vi "Invalid DLS Profile.vi"(0 "GEA2 Reference In":refnum<k24>, 1 "Shift To":enum16{"Spin", "Agitate"}(ring), 2 "Input Bit":T2, 5 "GEA Inputs":T4={"Source"=228, "Destination"=35} {"Destination" format="%.0x"; "Source" format="%.0x"}, 7 "Standalone?":bool, 11 "Error In":errorcluster, 12 "Action":enum16{"Lock", "Unlock"}(ring), 13 "Co-efficient Data":T1) -> (4 "GEA2 Reference Out":refnum<k24>, 10 "Report Text":string, 14 "Pass/Fail":bool, 15 "Error Out":errorcluster)   [LabVIEW 2016, in "TL27.lvlib"]
uses:
  Projects/TL27.lvlib
  C:/Automation/DLLs/PC Dot Net/GeaCommunication.dll
  Common/LabVIEW GEA2 Toolkit/LabVIEW_GEA2_Toolkit.lvlibp/type defs/Source_Destination.ctl
  Control/DLS ERD Data.ctl
  Valew Common/type defs/Drive Cycle Engine Request State.ctl
  Common/LabVIEW GEA2 Toolkit/LabVIEW_GEA2_Toolkit.lvlibp/type defs/ERD Read Data In.ctl
  Common/LabVIEW GEA2 Toolkit/LabVIEW_GEA2_Toolkit.lvlibp/type defs/Data Type.ctl
  Common/LabVIEW GEA2 Toolkit/LabVIEW_GEA2_Toolkit.lvlibp
panel:
  out "R1_DLS ERD Data":T3
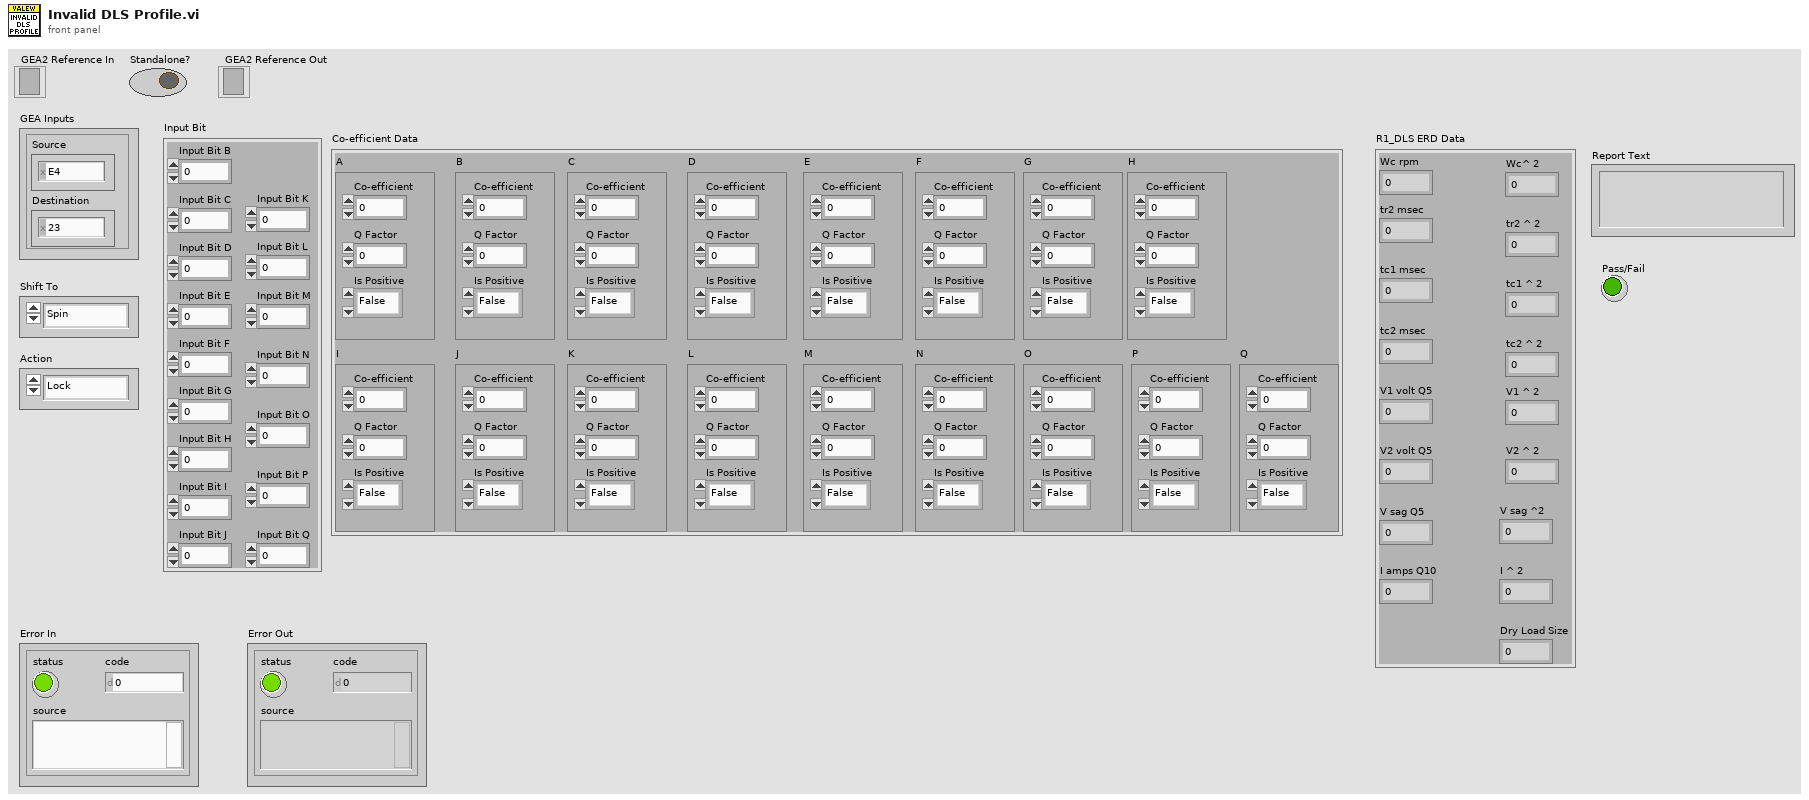
[diagram p1: front panel]
types:
  T1 = cluster{"A":cluster{"Co-efficient":dbl, "Q Factor":dbl, "Is Positive":enum16{"False", "True"}}, "B":cluster{"Co-efficient":dbl, "Q Factor":dbl, "Is Positive":enum16{"False", "True"}}, "C":cluster{"Co-efficient":dbl, "Q Factor":dbl, "Is Positive":enum16{"False", "True"}}, "D":cluster{"Co-efficient":dbl, "Q Factor":dbl, "Is Positive":enum16{"False", "True"}}, "E":cluster{"Co-efficient":dbl, "Q Factor":dbl, "Is Positive":enum16{"False", "True"}}, "F":cluster{"Co-efficient":dbl, "Q Factor":dbl, "Is Positive":enum16{"False", "True"}}, "G":cluster{"Co-efficient":dbl, "Q Factor":dbl, "Is Positive":enum16{"False", "True"}}, "H":cluster{"Co-efficient":dbl, "Q Factor":dbl, "Is Positive":enum16{"False", "True"}}, "I":cluster{"Co-efficient":dbl, "Q Factor":dbl, "Is Positive":enum16{"False", "True"}}, "J":cluster{"Co-efficient":dbl, "Q Factor":dbl, "Is Positive":enum16{"False", "True"}}, "K":cluster{"Co-efficient":dbl, "Q Factor":dbl, "Is Positive":enum16{"False", "True"}}, "L":cluster{"Co-efficient":dbl, "Q Factor":dbl, "Is Positive":enum16{"False", "True"}}, "M":cluster{"Co-efficient":dbl, "Q Factor":dbl, "Is Positive":enum16{"False", "True"}}, "N":cluster{"Co-efficient":dbl, "Q Factor":dbl, "Is Positive":enum16{"False", "True"}}, "O":cluster{"Co-efficient":dbl, "Q Factor":dbl, "Is Positive":enum16{"False", "True"}}, "P":cluster{"Co-efficient":dbl, "Q Factor":dbl, "Is Positive":enum16{"False", "True"}}, "Q":cluster{"Co-efficient":dbl, "Q Factor":dbl, "Is Positive":enum16{"False", "True"}}}
  T2 = cluster{"Input Bit B":dbl, "Input Bit C":dbl, "Input Bit D":dbl, "Input Bit E":dbl, "Input Bit F":dbl, "Input Bit G":dbl, "Input Bit H":dbl, "Input Bit I":dbl, "Input Bit J":dbl, "Input Bit K":dbl, "Input Bit L":dbl, "Input Bit M":dbl, "Input Bit N":dbl, "Input Bit O":dbl, "Input Bit P":dbl, "Input Bit Q":dbl}
  T3 = typedef "TL27.lvlib/DLS ERD Data.ctl" = cluster{"Wc rpm":dbl, "tr2 msec":dbl, "tc1 msec":dbl, "tc2 msec":dbl, "V1 volt Q5":dbl, "V2 volt Q5":dbl, "I amps Q10":dbl, "Wc^ 2":dbl, "tr2 ^ 2":dbl, "tc1 ^ 2":dbl, "tc2 ^ 2":dbl, "V1 ^ 2":dbl, "V2 ^ 2":dbl, "I ^ 2":dbl, "V sag Q5":dbl, "V sag ^2":dbl, "Dry Load Size":dbl}
  T4 = typedef "LabVIEW_GEA2_Toolkit.lvlibp/Source_Destination.ctl" = cluster{"Source":u8, "Destination":u8}
  T5 = enum16{"EQ (==)", "NE (!=)", "GT (>)", "LT (<)", "GE (>=)", "LE (<=)", "GTLT(> <)", "GELE (>= <=)", "GELT (>= <)", "GTLE (> <=)", "LTGT (< >)", "LEGE (<= >=)", "LEGT (<= >)", "LTGE (< >=)", "No Comparison"}
  T6 = typedef "LabVIEW_GEA2_Toolkit.lvlibp/ERD Read Data In.ctl" = cluster{"ERD Number":u16, "Data Type":T7}
  T7 = typedef "LabVIEW_GEA2_Toolkit.lvlibp/Data Type.ctl" = enum16{"string", "boolean", "uint8_t", "uint16_t", "uint32_t", "uint64_t", "int8_t", "int16_t", "int32_t", "int64_t"}
  T8 = typedef "TL27.lvlib/Drive Cycle Engine Request State.ctl" = enum16{"Start", "Stop", "Pause", "Resume", "Select"}
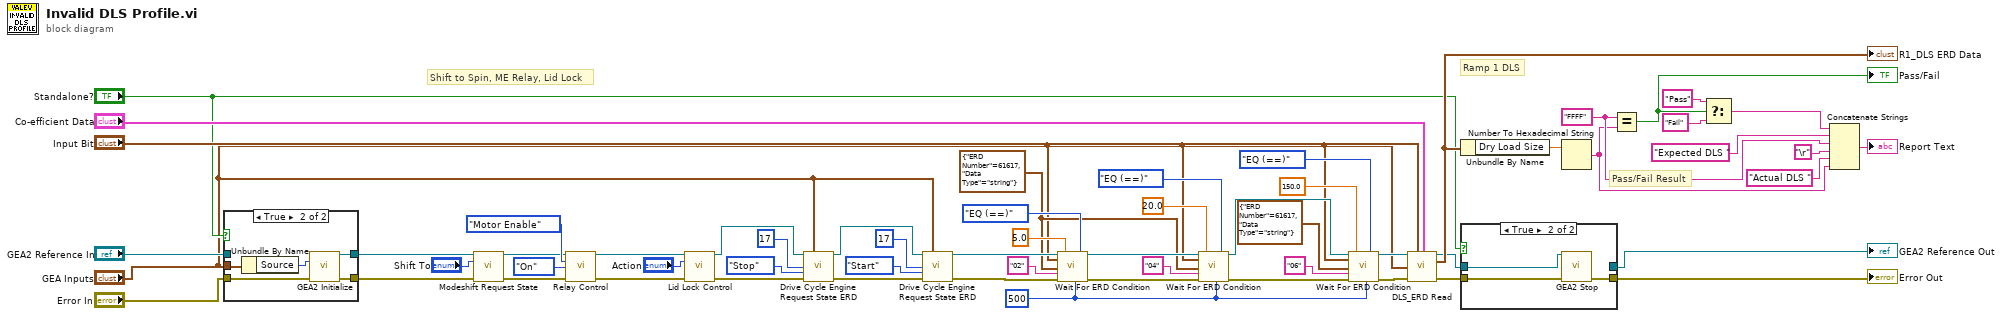
[diagram p0: block diagram]
diagram:
  w10 = "FFFF"
  w28 = u32 500 ("Loop Rate (ms)")
  w29 = T6 {"ERD Number"=61617, "Data Type"=enum."string"} ("ERD Read Data")
  # "Ramp 1 DLS"
  # "Pass/Fail Result"
  # "Shift to Spin, ME Relay, Lid Lock"
  n1 = case shown="True" "Standalone?" {
    tunnel: "GEA2 Reference In" -> [w62 _]
    tunnel: [w62 w67] -> w49
    tunnel: "Error In" -> [w61 w66]
    tunnel: [w61 w65] -> w47
    tunnel: "GEA Inputs" -> [_ w64]
    frame False {
    }
    frame True {
      n2 = Unbundle By Name(w64) -> ("Source"=w63:u8)
      n3 = call "GEA2 Initialize.vi"("Source Address"=w63, "error in"=w66) -> ("GEA2 Reference Out"=w67:refnum<k24>, "error out"=w65:errorcluster)  [unwired: 11 in, 1 out]
    }
  }
  n4 = call "Modeshift Request State.vi"("GEA2 Reference In"=w49, "Shift To"="Shift To", "Error In"=w47) -> ("GEA2 Reference Out"=w48:refnum<k24>, "Error Out"=w46:errorcluster)  [unwired: 9 in, 2 out]
  n5 = call "Relay Control.vi"("GEA2 Reference In"=w48, "Relay"=enum16{"Motor Enable", "Valve", "Both"}."Motor Enable", "State"=enum16{"On", "Off"}."On", "Error In"=w46) -> ("GEA2 Reference Out"=w56:refnum<k24>, "Error Out"=w54:errorcluster)  [unwired: 8 in, 2 out]
  n6 = call "Lid Lock Control.vi"("GEA2 Reference In"=w56, "Action"="Action", "Error In"=w54) -> ("GEA2 Reference Out"=w55:refnum<k24>, "Error Out"=w53:errorcluster)  [unwired: 9 in, 2 out]
  n7 = call "Drive Cycle Engine Request State ERD.vi"("GEA2 Reference In"=w55, "GEA Inputs"="GEA Inputs", "Cycle ID"=u8 17, "Drive Cycle Engine Request State"=Drive_Cycle_Engine_Request_State."Stop", "Error In"=w53) -> ("GEA2 Reference Out"=w44:refnum<k24>, "Error Out"=w43:errorcluster)  [unwired: 9 in]
  n8 = call "Drive Cycle Engine Request State ERD.vi"("GEA2 Reference In"=w44, "GEA Inputs"="GEA Inputs", "Cycle ID"=u8 17, "Drive Cycle Engine Request State"=Drive_Cycle_Engine_Request_State."Start", "Error In"=w43) -> ("GEA2 Reference Out"=w38:refnum<k24>, "Error Out"=w39:errorcluster)  [unwired: 9 in]
  n9 = call "Wait For ERD Condition.vi"("GEA2 Reference In"=w38, "GEA Inputs"="GEA Inputs", "ERD Read Data"=w29, "Expected Low"="02", "Error In"=w39, "Timeout (s)"=5.0, "Loop Rate (ms)"=w28, "Comparison"=T5."EQ (==)") -> ("GEA2 Reference Out"=w35:refnum<k24>, "Error Out"=w34:errorcluster)  [unwired: 7 in, 3 out]
  n10 = call "Wait For ERD Condition.vi"("GEA2 Reference In"=w35, "GEA Inputs"="GEA Inputs", "ERD Read Data"=w29, "Expected Low"="04", "Error In"=w34, "Timeout (s)"=20.0, "Loop Rate (ms)"=w28, "Comparison"=T5."EQ (==)") -> ("GEA2 Reference Out"=w30:refnum<k24>, "Error Out"=w6:errorcluster)  [unwired: 7 in, 3 out]
  n11 = call "Wait For ERD Condition.vi"("GEA2 Reference In"=w30, "GEA Inputs"="GEA Inputs", "ERD Read Data"=T6 {"ERD Number"=61617, "Data Type"=enum."string"}, "Expected Low"="06", "Error In"=w6, "Timeout (s)"=150.0, "Loop Rate (ms)"=w28, "Comparison"=T5."EQ (==)") -> ("GEA2 Reference Out"=w20:refnum<k24>, "Error Out"=w21:errorcluster)  [unwired: 7 in, 3 out]
  n12 = call "DLS_ERD Read.vi"("GEA2 Reference In"=w20, "Input Bit"="Input Bit", "Co-efficient Data"="Co-efficient Data", "GEA Inputs"="GEA Inputs", "Error In"=w21) -> ("GEA2 Reference Out"=w9:refnum<k24>, "DLS ERD Data"=w11:T3, "Error Out"=w8:errorcluster)  [unwired: 7 in, 1 out]
  "R1_DLS ERD Data" <- w11
  n13 = Unbundle By Name(w11) -> ("Dry Load Size"=w3:dbl)
  n14 = case shown="True" "Standalone?" {
    tunnel: [w69 w72] -> w25
    tunnel: w9 -> [w68 w71]
    tunnel: w8 -> [w69 w70]
    tunnel: [w68 _] -> w4
    frame False {
    }
    frame True {
      n15 = call "GEA2 Stop.vi"("GEA2 Reference In"=w71, "Error In"=w70) -> ("Error Out"=w72:errorcluster)  [unwired: 13 in]
    }
  }
  "GEA2 Reference Out" <- w4
  "Error Out" <- w25
  n16 = Number To Hexadecimal String(2:w3) -> (0:w2:string)  [unwired: 1 in]
  n17 = Equal?(x=w10, y=w2) -> (x = y?=w5:bool)
  "Pass/Fail" <- w5
  n18 = Select(t="Pass", s=w5, f="Fail") -> (s? t:f=w13:string)
  n19 = Concatenate Strings(w13, "Expected DLS " ("string"), w10, "\r", "Actual DLS " ("string"), w2) -> (→"Report Text":string)
